vi "Image Para Extract.vi"(8 "error in":errorcluster, 11 "Image Para":T1={"Marker"=enum."None", "Power(Amp)"=15, "set shutter(s)"=0.001, "Cube"=enum."1"} {"set shutter(s)" min=0.001 max=3.0 step=0.001; "Power(Amp)" min=15 max=100}) -> (0 "error out":errorcluster, 1 "Exposure(s)":dbl, 2 "Rotate U":i32, 3 "LED Control out":T3)   [LabVIEW 2019, in "LED.lvlib"]
uses:
  LED.lvlib
  Image Para.ctl
  Camera/Andor/SubVI/seletion.ctl
  Camera/Andor/Andor.lvlib
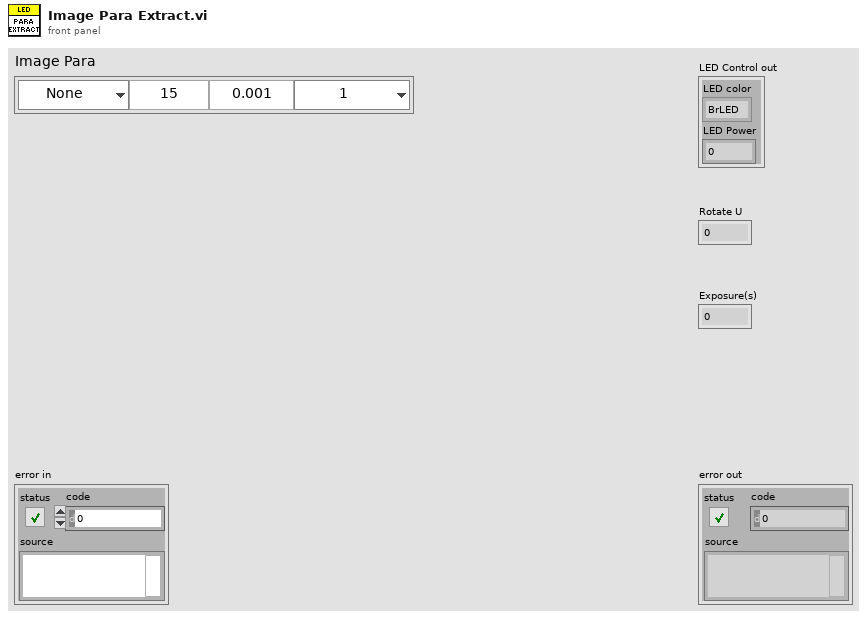
[diagram p1: front panel]
types:
  T1 = typedef "LED.lvlib/Image Para.ctl" = cluster{"Marker":T2, "Power(Amp)":u8, "set shutter(s)":dbl, "Cube":enum16{"1", "2", "3", "4", "5", "6", "7", "8"}}
  T2 = typedef "Andor.lvlib/seletion.ctl" = enum16{"None", "Red", "Green", "Blue", "UV", "Green Laser", "Blue-Red", "UV-Red", "BF", "UV-IR"}
  T3 = cluster{"LED color":enum32{"BrLED", "Blue", "Green", "Red", "UV"}, "LED Power":u8}
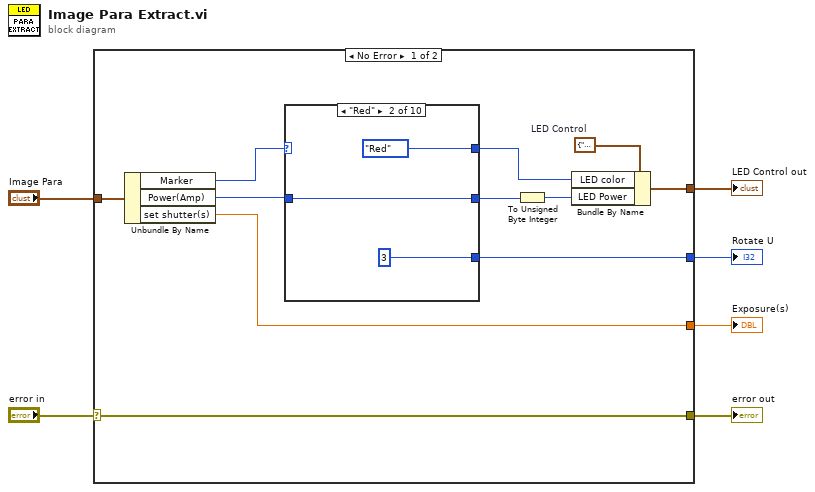
[diagram p0: block diagram]
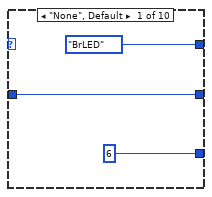
[diagram p2: hidden frame]
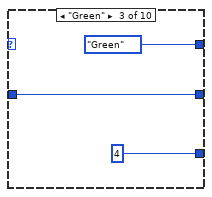
[diagram p3: hidden frame]
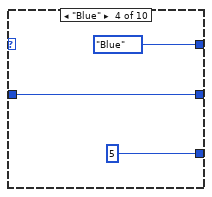
[diagram p4: hidden frame]
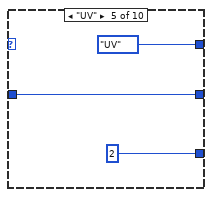
[diagram p5: hidden frame]
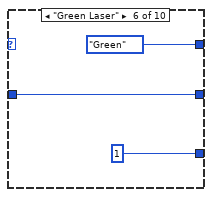
[diagram p6: hidden frame]
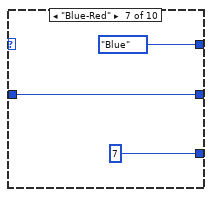
[diagram p7: hidden frame]
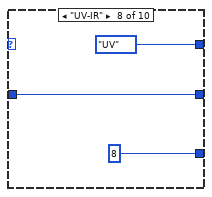
[diagram p8: hidden frame]
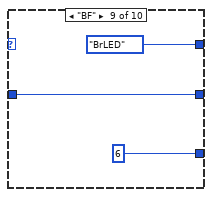
[diagram p9: hidden frame]
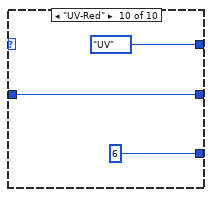
[diagram p10: hidden frame]
diagram:
  n1 = case shown="No Error" "error in" {
    selector: "error in" -> [w7 w48]
    tunnel: [w13 _] -> w6
    tunnel: [w12 _] -> w5
    tunnel: "Image Para" -> [w11 _]
    tunnel: [w8 _] -> w4
    tunnel: [w7 w48] -> w2
    frame No Error {
      w16 = T3 {"LED color"=enum."BrLED", "LED Power"=0}  # LED Control
      n2 = Unbundle By Name(w11) -> ("Marker"=w10:T2, "Power(Amp)"=w9:u8, "set shutter(s)"=w8:dbl)
      n3 = case shown="\"Red\"" w10 {
        tunnel: [w20 w23 w26 w29 w32 w35 w38 w41 w44 w47] -> w15
        tunnel: w9 -> [w20 w23 w26 w29 w32 w35 w38 w41 w44 w47]
        tunnel: [enum32{"BrLED", "Blue", "Green", "Red", "UV"}."BrLED" ("LED color") enum32{"BrLED", "Blue", "Green", "Red", "UV"}."Red" ("LED color") enum32{"BrLED", "Blue", "Green", "Red", "UV"}."Green" ("LED color") enum32{"BrLED", "Blue", "Green", "Red", "UV"}."Blue" ("LED color") enum32{"BrLED", "Blue", "Green", "Red", "UV"}."UV" ("LED color") enum32{"BrLED", "Blue", "Green", "Red", "UV"}."Green" ("LED color") enum32{"BrLED", "Blue", "Green", "Red", "UV"}."Blue" ("LED color") enum32{"BrLED", "Blue", "Green", "Red", "UV"}."UV" ("LED color") enum32{"BrLED", "Blue", "Green", "Red", "UV"}."BrLED" ("LED color") enum32{"BrLED", "Blue", "Green", "Red", "UV"}."UV" ("LED color")] -> w14
        tunnel: [6 3 4 5 2 1 7 8 6 6] -> w13
        frame "None", Default {
        }
        frame "Red" {
        }
        frame "Green" {
        }
        frame "Blue" {
        }
        frame "UV" {
        }
        frame "Green Laser" {
        }
        frame "Blue-Red" {
        }
        frame "UV-IR" {
        }
        frame "BF" {
        }
        frame "UV-Red" {
        }
      }
      n4 = To Unsigned Byte Integer(number=w15) -> (unsigned 8bit integer=w17:u8)
      n5 = Bundle By Name(cluster=w16, "LED color"=w14, "LED Power"=w17) -> (w12:T3)
    }
    frame Error {
    }
  }
  "Rotate U" <- w6
  "LED Control out" <- w5
  "Exposure(s)" <- w4
  "error out" <- w2
